vi "CloseDOSession.vi"(8 "error in (no error)":errorcluster, 10 "gRPCid":T5, 11 "DIOSessions In":T1={"Array of DI Sessions"=[], "Array of DO Sessions"=[], "Stream ReadDI"={"gRPCid ReadDI"=0, "DISessionName"="", "Stream Status ReadDI"=FALSE, "Async Stop ReadDI Queue"=refnum, "DI Task"="", "ms to wait"=500}}) -> (0 "error out":errorcluster, 3 "DIOSessions Out":T1={"Array of DI Sessions"=[], "Array of DO Sessions"=[], "Stream ReadDI"={"gRPCid ReadDI"=0, "DISessionName"="", "Stream Status ReadDI"=FALSE, "Async Stop ReadDI Queue"=refnum, "DI Task"="", "ms to wait"=500}})   [LabVIEW 2019, in "ctet_dio_User Library.lvlib"]
uses:
  ctet_dio_User Library.lvlib
  Servers/ctet_dio/gRPC lvSupport/Server API/typeDefs/grpcId.ctl
  Types/DIOSessions.ctl
  Types/DISession.ctl
  Types/DOSession.ctl
  Types/StreamReadDI.ctl
  Servers/ctet_dio/ctet_dio Class/RPC Messages/measurementservice_DOCloseSessionResponse/measurementservice_DOCloseSessionResponse_Data.ctl
  Servers/ctet_dio/ctet_dio Class/RPC Messages/measurementservice_ErrorOut/measurementservice_ErrorOut_Data.ctl
  Servers/ctet_dio/ctet_dio Class/ctet_dio.lvclass
  Servers/ctet_dio/gRPC lvSupport/gprc-lvsupport.lvlib
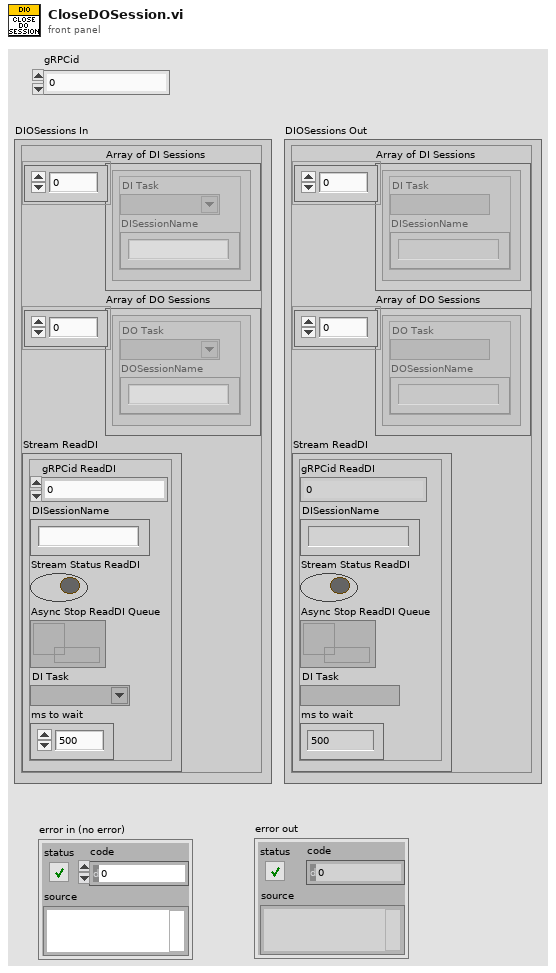
[diagram p1: front panel]
types:
  T1 = typedef "ctet_dio_User Library.lvlib/DIOSessions.ctl" = cluster{"Array of DI Sessions":T2[], "Array of DO Sessions":T3[], "Stream ReadDI":T4}
  T2 = typedef "ctet_dio_User Library.lvlib/DISession.ctl" = cluster{"DI Task":refnum<k21>, "DISessionName":string}
  T3 = typedef "ctet_dio_User Library.lvlib/DOSession.ctl" = cluster{"DO Task":refnum<k21>, "DOSessionName":string}
  T4 = typedef "ctet_dio_User Library.lvlib/StreamReadDI.ctl" = cluster{"gRPCid ReadDI":T5, "DISessionName":string, "Stream Status ReadDI":bool, "Async Stop ReadDI Queue":refnum<queue>, "DI Task":refnum<k21>, "ms to wait":u32}
  T5 = typedef "ctet_dio.lvlib/gprc-lvsupport.lvlib/grpcId.ctl" = u64
  T6 = typedef "ctet_dio.lvlib/ctet_dio.lvclass/measurementservice_ErrorOut_Data.ctl" = cluster{"errCode":i64, "errMessage":string}
  T7 = typedef "ctet_dio.lvlib/ctet_dio.lvclass/measurementservice_DOCloseSessionResponse_Data.ctl" = cluster{"error":T6}
  T8 = typedef "ctet_dio.lvlib/ctet_dio.lvclass/measurementservice_DOCloseSessionRequest_Data.ctl" = cluster{"DOSessionName":string}
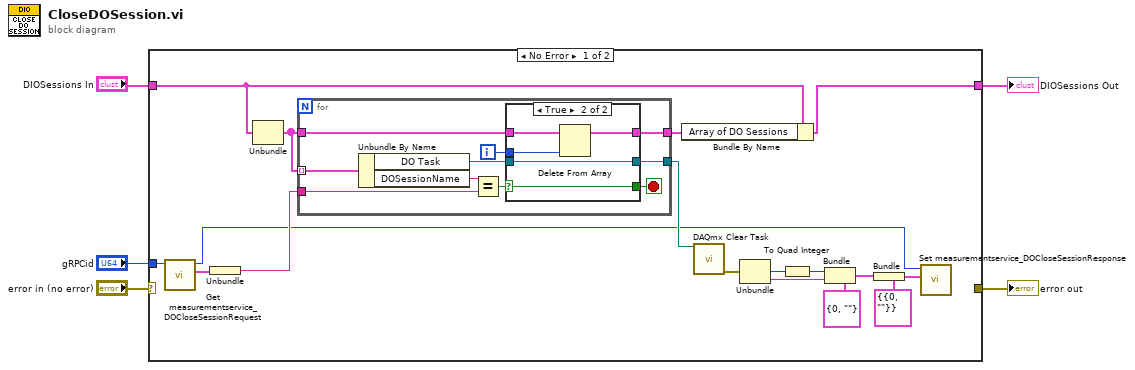
[diagram p0: block diagram]
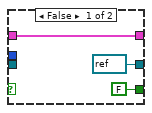
[diagram p2: hidden frame]
diagram:
  n1 = case shown="No Error" "error in (no error)" {
    selector: "error in (no error)" -> [_ w42]
    tunnel: [_ w42] -> w5
    tunnel: "gRPCid" -> [w13 _]
    tunnel: "DIOSessions In" -> [w19 w41]
    tunnel: [w18 w41] -> w1
    frame No Error {
      n2 = call "Get measurementservice_DOCloseSessionRequest.vi"("gRPCid"=w13) -> ("Message Data"=w12:T8, "gRPCid out"=w8:T5)  [unwired: 8 in, 1 out]
      n3 = Unbundle(w12) -> ("DOSessionName"=w17:string)
      n4 = Unbundle(w19) -> ("Array of DO Sessions"=w11:T3[])  [unwired: 2 out]
      n5 = for {
        tunnel: w11 -> [w27] mode=indexing
        tunnel: w17 -> [w32]
        tunnel: [w28] -> w21
        tunnel: w11 -> [w26]
        tunnel: [w25] -> w20
        i -> [w23]
        stop <- w30 stop-if-true
        n6 = Unbundle By Name(w27) -> ("DO Task"=w29:refnum<k21>, "DOSessionName"=w24:string)
        n7 = Equal?(x=w24, y=w32) -> (x = y?=w31:bool)
        n8 = case shown="True" w31 {
          selector: w31 -> [_ w40]
          tunnel: [FALSE w40] -> w30
          tunnel: w29 -> [_ w38]
          tunnel: [refnum<k21> refnum ("DI Task") w38] -> w28
          tunnel: w26 -> [w33 w39]
          tunnel: [w33 w36] -> w25
          tunnel: w23 -> [_ w37]
          frame False {
          }
          frame True {
            n9 = Delete From Array(array=w39, index=w37) -> (array with subset deleted=w36:T3[])  [unwired: 1 in, 1 out]
          }
        }
      }
      n10 = Bundle By Name(cluster=w19, "Array of DO Sessions"=w20) -> (w18:T1)
      n11 = call <vilib>:"DAQmx Clear Task.vi"("task in"=w21) -> ("error out"=w22:errorcluster)  [unwired: 14 in]
      n12 = Unbundle(w22) -> ("code"=w15:i32, "source"=w16:string)  [unwired: 1 out]
      n13 = To Quad Integer(1:w15) -> (0:w14:i64)
      n14 = Bundle(cluster=T6 {"errCode"=0, "errMessage"=""} ("error"), "errCode"=w14, "errMessage"=w16) -> (w6:T6)
      n15 = Bundle(cluster=T7 {"error"={"errCode"=0, "errMessage"=""}} ("measurementservice_DOCloseSessionResponse_Data"), "error"=w6) -> (w9:T7)
      n16 = call "Set measurementservice_DOCloseSessionResponse.vi"("Message Data"=w9, "gRPCid"=w8) -> ()  [unwired: 9 in, 1 out]
    }
    frame Error {
    }
  }
  "error out" <- w5
  "DIOSessions Out" <- w1
